vi "onProcessResults.vi"(8 "error in (no error)":errorcluster, 11 "Pips.TestResults in":refnum<class "Pips.TestResults.lvclass">) -> (0 "error out":errorcluster, 3 "Pips.TestResults out":refnum<class "Pips.TestResults.lvclass">)   [LabVIEW 2021, in "Banana.Caraya.lvlib" / "Pips.TestResults.lvclass"]
uses:
  Pips.TestResults.lvclass
  Pips.TestResults.lvclass/Pips.TestResults.ctl
  <vilib>/addons/_JKI Toolkits/Caraya/classes/Test Result/Test Result.lvclass
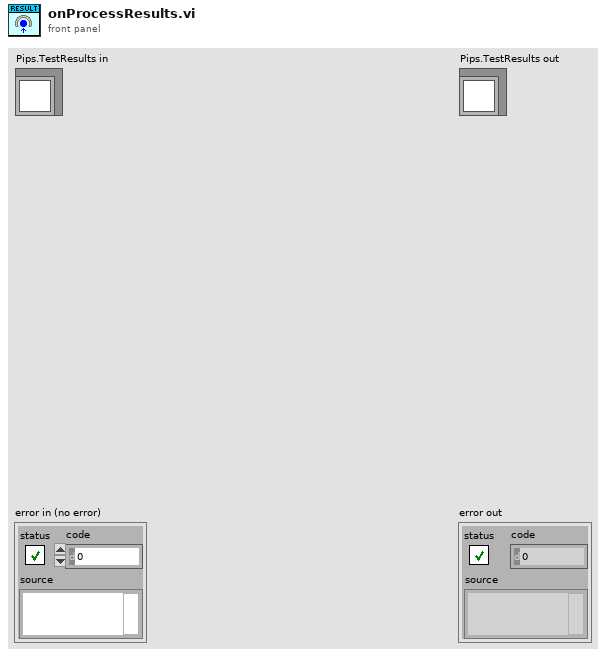
[diagram p1: front panel]
types:
  T1 = cluster{"passed":set{string}, "failed":set{string}, "skipped":set{string}}
  T2 = typedef "Caraya.lvlib/Test Result.lvclass/Assert Event Data (Extended).ctl" = cluster{"name":string, "passed":bool, "call-chain":string[], "test-error":errorcluster, "timestamp":timestamp, "assert-id":string, "test-id":string, "time":dbl, "message":string, "properties":variant, "measurements":variant, "user-defined":variant}
  T3 = typedef "Caraya.lvlib/Test Result.lvclass/Test Node (Extended).ctl" = cluster{"Test Registration":T4, "Defined":bool, "Passed":bool, "properties":variant}
  T4 = typedef "Caraya.lvlib/Test Result.lvclass/Test Registration Data.ctl" = cluster{"Name":string, "Call Chain":string[], "Time Stamp":timestamp, "Test ID":string, "Caller ID":string}
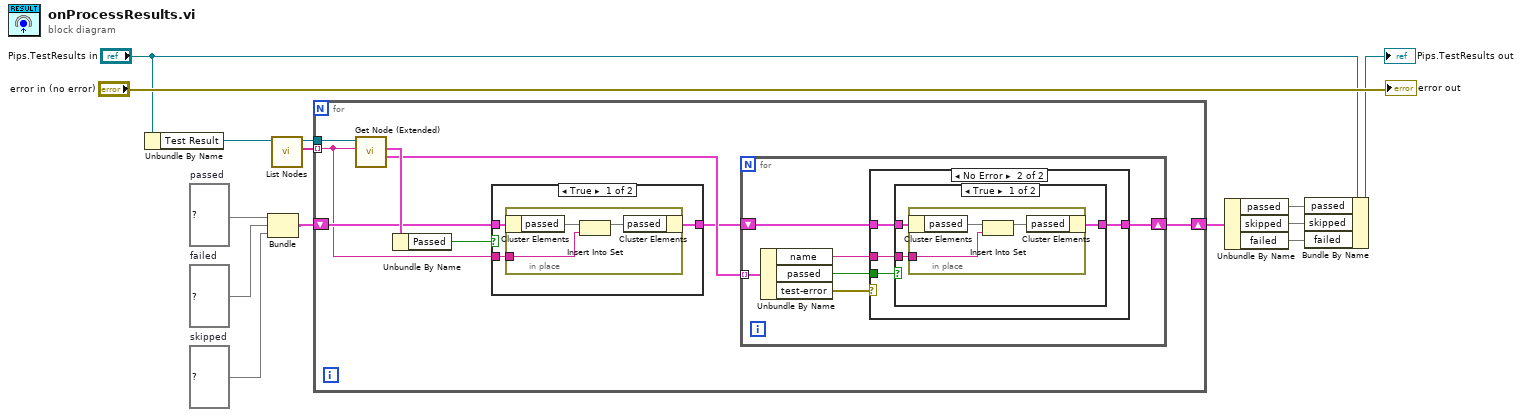
[diagram p0: block diagram]
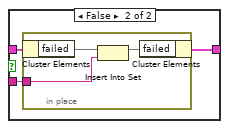
[diagram p2: hidden frame]
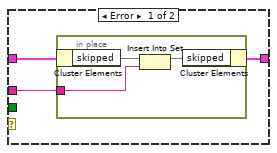
[diagram p3: hidden frame]
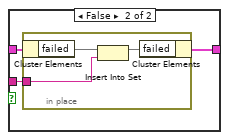
[diagram p4: hidden frame]
diagram:
  w9 = set{string} {}  # failed
  w8 = set{string} {}  # skipped
  w10 = set{string} {}  # passed
  n1 = Unbundle By Name("Pips.TestResults in") -> ("Test Result"=w11:refnum<class "Test Result.lvclass">)
  n2 = Bundle("passed"=w10, "failed"=w9, "skipped"=w8) -> (w7:T1)  [unwired: 1 in]
  n3 = call <vilib>:"List Nodes.vi"("Test Result in"=w11) -> ("Nodes"=w13:string[], "Test Result out"=w14:refnum<class "Test Result.lvclass">)  [unwired: 8 in, 1 out]
  n4 = for {
    tunnel: w14 -> [w22]
    tunnel: w13 -> [w17] mode=indexing
    shift-right: [w15] -> w4
    shift-left: w7 -> [w19]
    n5 = call <vilib>:"Get Node (Extended).vi"("Node"=w17, "Test Result in"=w22) -> ("Assertions"=w20:T2[], "Test Node"=w21:T3)  [unwired: 4 in, 4 out]
    n6 = Unbundle By Name(w21) -> ("Passed"=w18:bool)
    n7 = case shown="True" w18 {
      tunnel: w19 -> [w25 w31]
      tunnel: [w24 w30] -> w16
      tunnel: w17 -> [w23 w29]
      frame True {
        n8 = in-place {
          in-place-border: w23 -> [w26]
          n9 = in-place-cluster #1(w25) -> ("passed"=w28:set{string})
          n10 = Insert Into Set(10:w26, 11:w28) -> (3:w27:set{string})  [unwired: 1 out]
          n11 = in-place-cluster #1("passed"=w27) -> (w24:T1)
        }
      }
      frame False {
        n12 = in-place {
          in-place-border: w29 -> [w32]
          n13 = in-place-cluster #2(w31) -> ("failed"=w34:set{string})
          n14 = Insert Into Set(10:w32, 11:w34) -> (3:w33:set{string})  [unwired: 1 out]
          n15 = in-place-cluster #2("failed"=w33) -> (w30:T1)
        }
      }
    }
    n16 = for {
      tunnel: w20 -> [w40] mode=indexing
      shift-right: [w35] -> w15
      shift-left: w16 -> [w38]
      n17 = Unbundle By Name(w40) -> ("name"=w37:string, "passed"=w36:bool, "test-error"=w39:errorcluster)
      n18 = case shown="No Error" w39 {
        tunnel: w38 -> [w43 w49]
        tunnel: [w42 w50] -> w35
        tunnel: w37 -> [w41 w47]
        tunnel: w36 -> [_ w48]
        frame Error {
          n19 = in-place {
            in-place-border: w41 -> [w44]
            n20 = in-place-cluster #3(w43) -> ("skipped"=w46:set{string})
            n21 = Insert Into Set(10:w44, 11:w46) -> (3:w45:set{string})  [unwired: 1 out]
            n22 = in-place-cluster #3("skipped"=w45) -> (w42:T1)
          }
        }
        frame No Error {
          n23 = case shown="True" w48 {
            tunnel: w49 -> [w53 w59]
            tunnel: [w52 w58] -> w50
            tunnel: w47 -> [w51 w57]
            frame True {
              n24 = in-place {
                in-place-border: w51 -> [w54]
                n25 = in-place-cluster #4(w53) -> ("passed"=w56:set{string})
                n26 = Insert Into Set(10:w54, 11:w56) -> (3:w55:set{string})  [unwired: 1 out]
                n27 = in-place-cluster #4("passed"=w55) -> (w52:T1)
              }
            }
            frame False {
              n28 = in-place {
                in-place-border: w57 -> [w60]
                n29 = in-place-cluster #5(w59) -> ("failed"=w62:set{string})
                n30 = Insert Into Set(10:w60, 11:w62) -> (3:w61:set{string})  [unwired: 1 out]
                n31 = in-place-cluster #5("failed"=w61) -> (w58:T1)
              }
            }
          }
        }
      }
    }
  }
  n32 = Unbundle By Name(w4) -> ("passed"=w3:set{string}, "skipped"=w2:set{string}, "failed"=w1:set{string})
  n33 = Bundle By Name(cluster="Pips.TestResults in", "passed"=w3, "skipped"=w2, "failed"=w1) -> (→"Pips.TestResults out":refnum<class "Pips.TestResults.lvclass">)
  "error out" <- "error in (no error)"
